vi "电机定位（test）.vi"(4 "细分设置":dbl=8.0, 6 "电机急停":bool, 7 "等待时间(ms)":u32=40, 8 "精度":dbl=0.001, 9 "X":dbl, 11 "VISA I":refnum<visa-resource-name>) -> (1 "X":dbl, 3 "VISA O":refnum<visa-resource-name>)   [LabVIEW 2016]
panel:
  out "数值":i32
  in  "确定":bool
  in  "ESC":bool
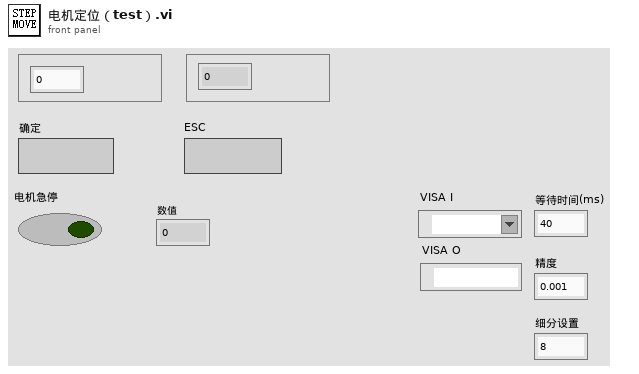
[diagram p1: front panel]
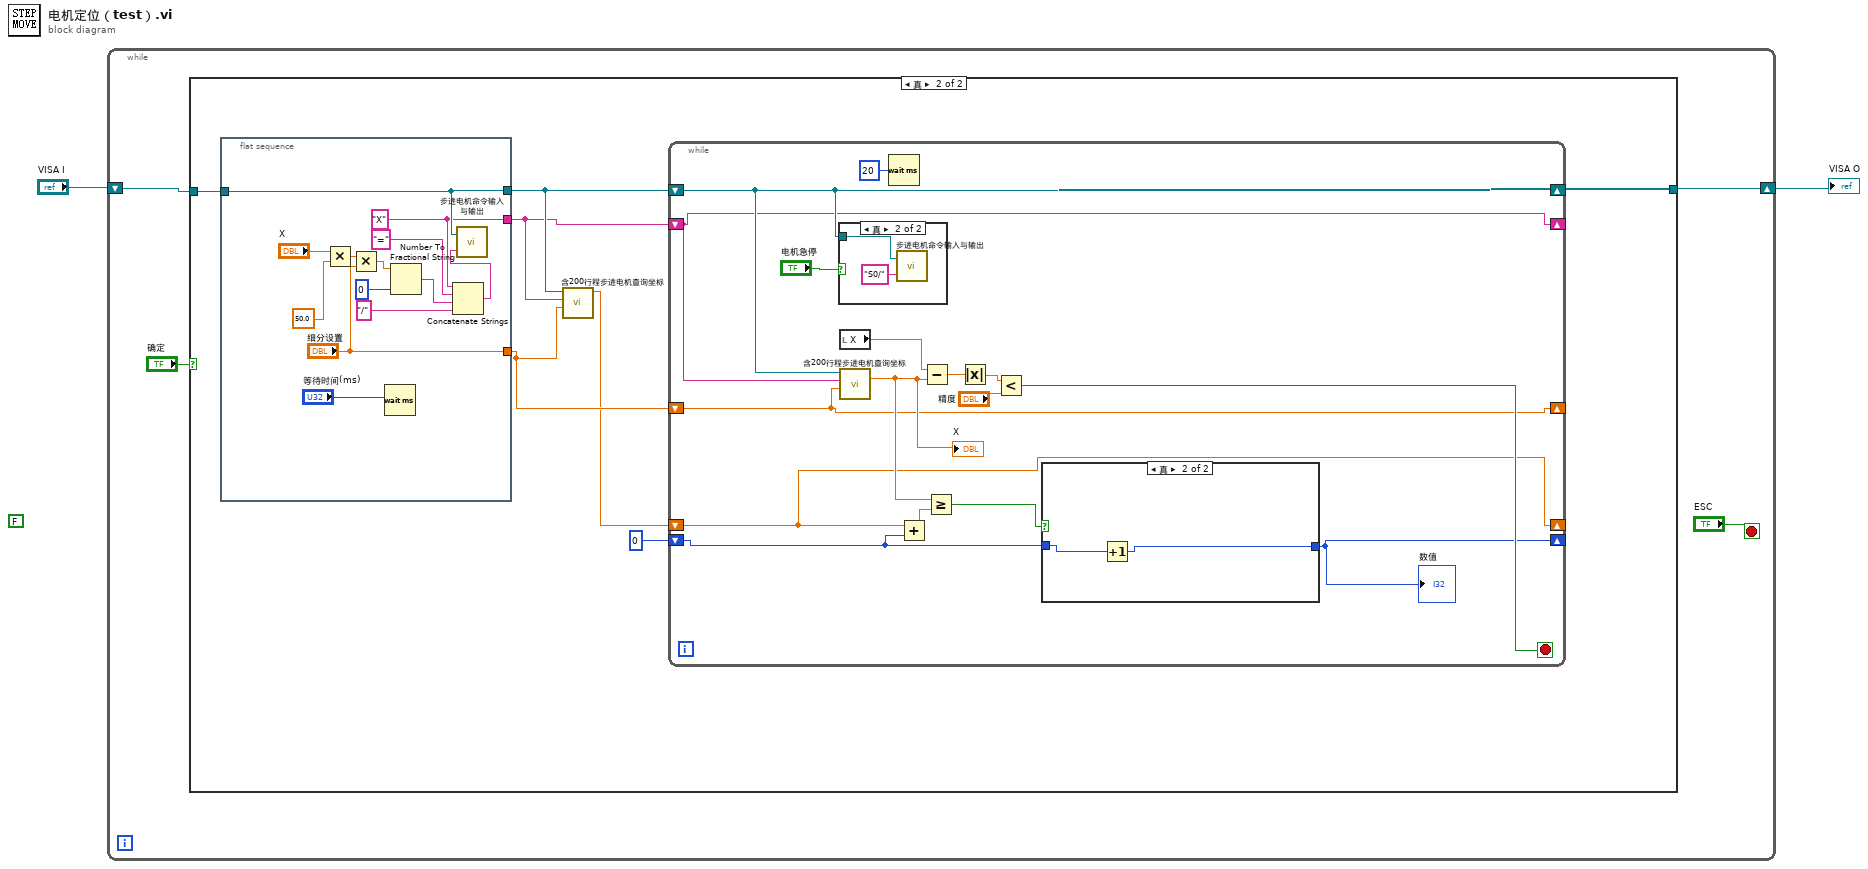
[diagram p0: block diagram]
diagram:
  (unwired) FALSE
  n1 = while {
    shift-right: [w5] -> w2
    shift-left: "VISA I" -> [w6]
    stop <- "ESC" stop-if-true
    n2 = case shown="真" "确定" {
      tunnel: w6 -> [w7 w14]
      tunnel: [w7 w13] -> w5
      frame False {
      }
      frame True {
        n3 = flat-sequence {
          tunnel: w14 -> [w40]
          tunnel: [w40] -> w11
          tunnel: ["细分设置"] -> w9
          tunnel: [w37] -> w10
          frame #0 {
            w37 = "X"
            n4 = Multiply(x="X", y=50.0 ("x")) -> (x*y=w43:dbl)
            n5 = Multiply(x=w43, y="细分设置") -> (x*y=w48:dbl)
            n6 = Wait (ms)(milliseconds to wait="等待时间(ms)") -> ()  [unwired: 1 out]
            n7 = Number To Fractional String(number=w48, precision (6)=i16 0 ("精度(6)")) -> (F-format string=w46:string)  [unwired: 2 out]
            n8 = Concatenate Strings(w37, "=" ("字符串"), w46, "/" ("字符串")) -> (w42:string)
            n9 = call "步进电机命令输入与输出.vi"("输入字符串"=w42, "串口通信端口"=w40) -> ()  [unwired: 1 out]
          }
        }
        n10 = call "含200行程步进电机查询坐标.vi"("细分设置"=w9, "查询坐标轴"=w10, "串口通信端口"=w11) -> ("坐标(mm)"=w8:dbl)  [unwired: 8 in]
        n11 = while {
          shift-right: [w28] -> w13
          shift-left: w11 -> [w28]
          shift-right: [w23] -> _
          shift-left: 0 -> [w21]
          shift-right: [w16] -> _
          shift-left: w8 -> [w16]
          shift-right: [w15] -> _
          shift-left: w9 -> [w15]
          shift-right: [w17] -> _
          shift-left: w10 -> [w17]
          stop <- w26 stop-if-true
          n12 = case shown="真" "电机急停" {
            tunnel: w28 -> [_ w34]
            frame False {
            }
            frame True {
              n13 = call "步进电机命令输入与输出.vi"("输入字符串"="S0/", "串口通信端口"=w34) -> ()  [unwired: 1 out]
            }
          }
          n14 = local read "X"() -> (w22:dbl)
          n15 = call "含200行程步进电机查询坐标.vi"("细分设置"=w15, "查询坐标轴"=w17, "串口通信端口"=w28) -> ("坐标(mm)"=w19:dbl)  [unwired: 8 in]
          "X" <- w19
          n16 = Wait (ms)(milliseconds to wait=u32 20 ("等待时间（毫秒）")) -> ()  [unwired: 1 out]
          n17 = Add(x=w16, y=w21) -> (x+y=w20:dbl)
          n18 = Subtract(x=w22, y=w19) -> (x-y=w30:dbl)
          n19 = Greater Or Equal?(x=w19, y=w20) -> (x >= y?=w18:bool)
          n20 = Absolute Value(x=w30) -> (abs(x)=w29:dbl)
          n21 = Less?(x=w29, y="精度") -> (x < y?=w26:bool)
          n22 = case shown="真" w18 {
            tunnel: w21 -> [w31 w33]
            tunnel: [w31 w32] -> w23
            frame False {
            }
            frame True {
              n23 = Increment(x=w33) -> (x+1=w32:i32)
            }
          }
          "数值" <- w23
        }
      }
    }
  }
  "VISA O" <- w2
